vi "Tanh.vi"(2 "Z":dbl[][](array[numeric])) -> (0 "Exp(Z)":dbl[][](array[numeric]))   [LabVIEW 2020]
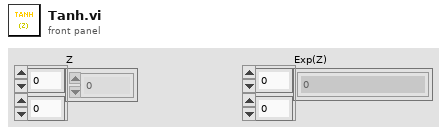
[diagram p1: front panel]
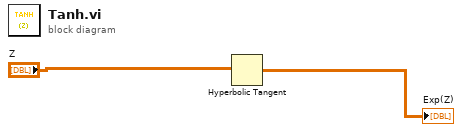
[diagram p0: block diagram]
diagram:
  n1 = Hyperbolic Tangent(1:"Z") -> (0:→"Exp(Z)":dbl[][])
